vi "BetterErrorText.vi"(8 "error in (no error)":errorcluster, 11 "Python":T2) -> (2 "Disabled":T1(ring), 3 "Python out":T2)   [LabVIEW 2022 SP3]
uses:
  PythonCtrl.ctl
  Processors.ctl
  <vilib>/Platform/browser.llb/Open URL in Default Browser (string).vi
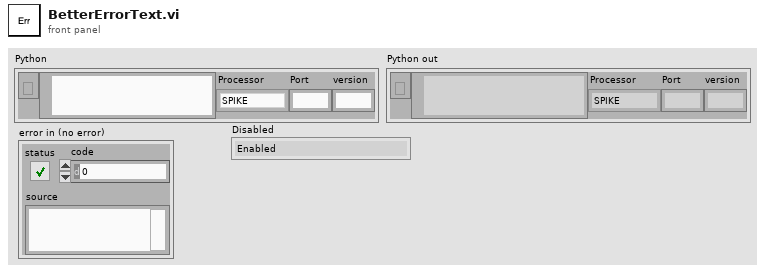
[diagram p1: front panel]
types:
  T1 = enum8{"Enabled", "Disabled", "Disabled and Grayed Out"}
  T2 = typedef "PythonCtrl.ctl" = cluster{"session":refnum<k35>, "PyPath":path, "Processor":T3, "Port":string, "version":string}
  T3 = typedef "Processors.ctl" = enum16{"SPIKE", "Pi", "Pi_ssh", "OpenMV", "Dunio"}
  T4 = enum16{"Left Button", "Center Button", "Right Button", "Window Close"}
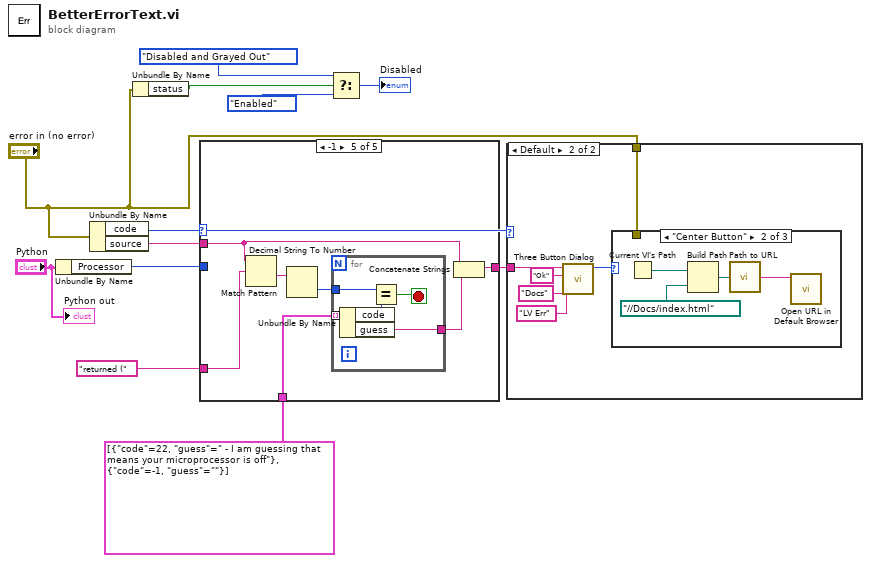
[diagram p0: block diagram]
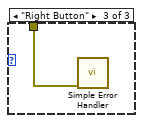
[diagram p4: hidden frame]
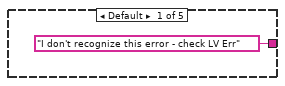
[diagram p5: hidden frame]
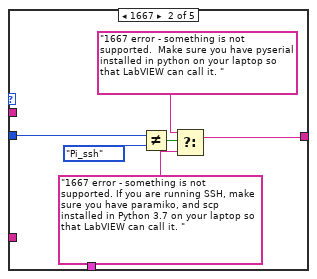
[diagram p6: hidden frame]
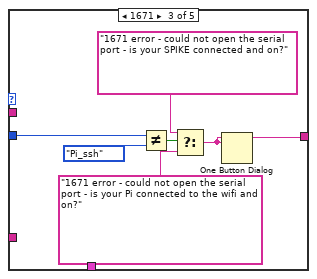
[diagram p7: hidden frame]
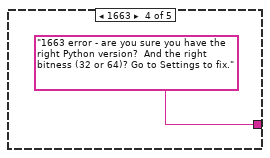
[diagram p8: hidden frame]
diagram:
  n1 = Unbundle By Name("Python") -> ("Processor"=w11:T3)
  n2 = Unbundle By Name("error in (no error)") -> ("code"=w3:i32, "source"=w10:string)
  n3 = Unbundle By Name("error in (no error)") -> ("status"=w6:bool)
  n4 = case shown="-1" w3 {
    tunnel: w11 -> [_ w17 w23 _ _]
    tunnel: w10 -> [_ _ _ _ w29]
    tunnel: ["I don't recognize this error - check LV Err" ("message") w14 w20 "1663 error - are you sure you have the right Python version?  And the right bitness (32 or 64)? Go to Settings to fix." ("message") w27] -> w5
    tunnel: "returned (" ("regular expression") -> [_ _ _ _ w33]
    tunnel: cluster{"code":i32, "guess":string}[] [{"code"=22, "guess"=" - I am guessing that means your microprocessor is off"}, {"code"=-1, "guess"=""}] -> [_ _ _ _ w31]
    frame Default {
    }
    frame 1667 {
      n5 = Not Equal?(x=w17, y=enum16{"SPIKE", "Pi", "Pi_ssh"}."Pi_ssh" ("Processor")) -> (x != y?=w19:bool)
      n6 = Select(t="1667 error - something is not supported.  Make sure you have pyserial installed in python on your laptop so that LabVIEW can call it. " ("message"), s=w19, f="1667 error - something is not supported. If you are running SSH, make sure you have paramiko, and scp installed in Python 3.7 on your laptop so that LabVIEW can call it. " ("message")) -> (s? t:f=w14:string)
    }
    frame 1671 {
      n7 = Not Equal?(x=w23, y=enum16{"SPIKE", "Pi", "Pi_ssh"}."Pi_ssh" ("Processor")) -> (x != y?=w25:bool)
      n8 = Select(t="1671 error - could not open the serial port - is your SPIKE connected and on?" ("message"), s=w25, f="1671 error - could not open the serial port - is your Pi connected to the wifi and on?" ("message")) -> (s? t:f=w20:string)
      n9 = One Button Dialog(message=w20) -> ()  [unwired: 1 in, 1 out]
    }
    frame 1663 {
    }
    frame -1 {
      n10 = Match Pattern(string=w29, regular expression=w33) -> (after substring=w32:string)  [unwired: 1 in, 3 out]
      n11 = Decimal String To Number(string=w32) -> (number=w30:i32)  [unwired: 2 in, 1 out]
      n12 = for {
        tunnel: w31 -> [w38] mode=indexing
        tunnel: w30 -> [w37]
        tunnel: [w34] -> w28
        stop <- w35 stop-if-true
        n13 = Unbundle By Name(w38) -> ("code"=w36:i32, "guess"=w34:string)
        n14 = Equal?(x=w37, y=w36) -> (x = y?=w35:bool)
      }
      n15 = Concatenate Strings(w29, w28) -> (w27:string)
    }
  }
  n16 = Select(t=T1."Disabled and Grayed Out" ("Disabled"), s=w6, f=T1."Enabled" ("Disabled")) -> (s? t:f=→"Disabled":T1)
  n17 = case shown="Default" w3 {
    tunnel: w5 -> [_ w44]
    tunnel: "error in (no error)" -> [_ w39]
    frame 0 {
    }
    frame Default {
      n18 = call <vilib>:"Three Button Dialog.vi"("Right Button Text (\"Cancel\")"="LV Err" ("Right Button Text (\"Cancel\")"), "Center Button Text (\"No\")"="Docs" ("Center Button Text (\"No\")"), "Left Button Text (\"Yes\")"="Ok" ("Left Button Text (\"Yes\")"), "message"=w44) -> ("Which Button?"=w40:T4)  [unwired: 7 in]
      n19 = case shown="\"Center Button\"" w40 {
        tunnel: w39 -> [_ _ w49]
        frame "Left Button", Default {
        }
        frame "Center Button" {
          n20 = Current VI's Path() -> (path=w48:path)
          n21 = Build Path(base path=w48, name or relative path=path "../../Docs/index.html") -> (appended path=w45:path)
          n22 = call <vilib>:"Path to URL.vi"("path"=w45) -> ("url"=w46:string)
          n23 = call-poly <vilib>:"Open URL in Default Browser.vi"("URL"=w46) -> ()  [unwired: 5 in, 2 out]
        }
        frame "Right Button" {
          n24 = call <vilib>:"Simple Error Handler.vi"("error in (no error)"=w49) -> ()  [unwired: 4 in, 5 out]
        }
      }
    }
  }
  "Python out" <- "Python"
